vi "Prompt for Step.vi"(8 "error in (no error)":errorcluster, 10 "Subpanel Ref":refnum<vi>, 11 "Step in":refnum<class "Step.lvclass">) -> (0 "error out":errorcluster, 3 "Step out":refnum<class "Step.lvclass">)   [LabVIEW 2020, in "MacroAssert.lvlib" / "Step.lvclass"]
doc: "Displays its own window into <B>Subpanel Ref</B> for the user to enter a macro step."
uses:
  Step.lvclass
  <vilib>/Utility/inputDevices.llb/closeMouse.vi
  Support/Get Control Reference by Label (0D STR).vi
  SubVIs/FaKI State Machine/FaKI State Machine.lvlib
  MacroAssert.lvlib
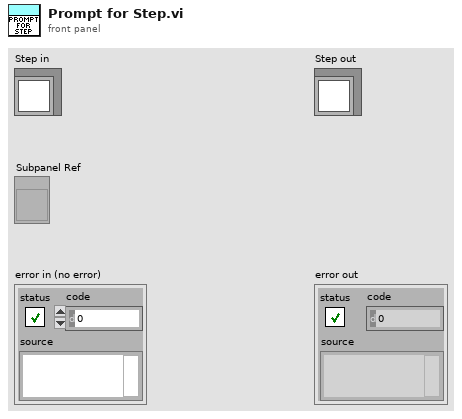
[diagram p1: front panel]
types:
  T1 = enum32{"Invalid", "Standard", "Closed", "Hidden", "Minimized", "Maximized"}
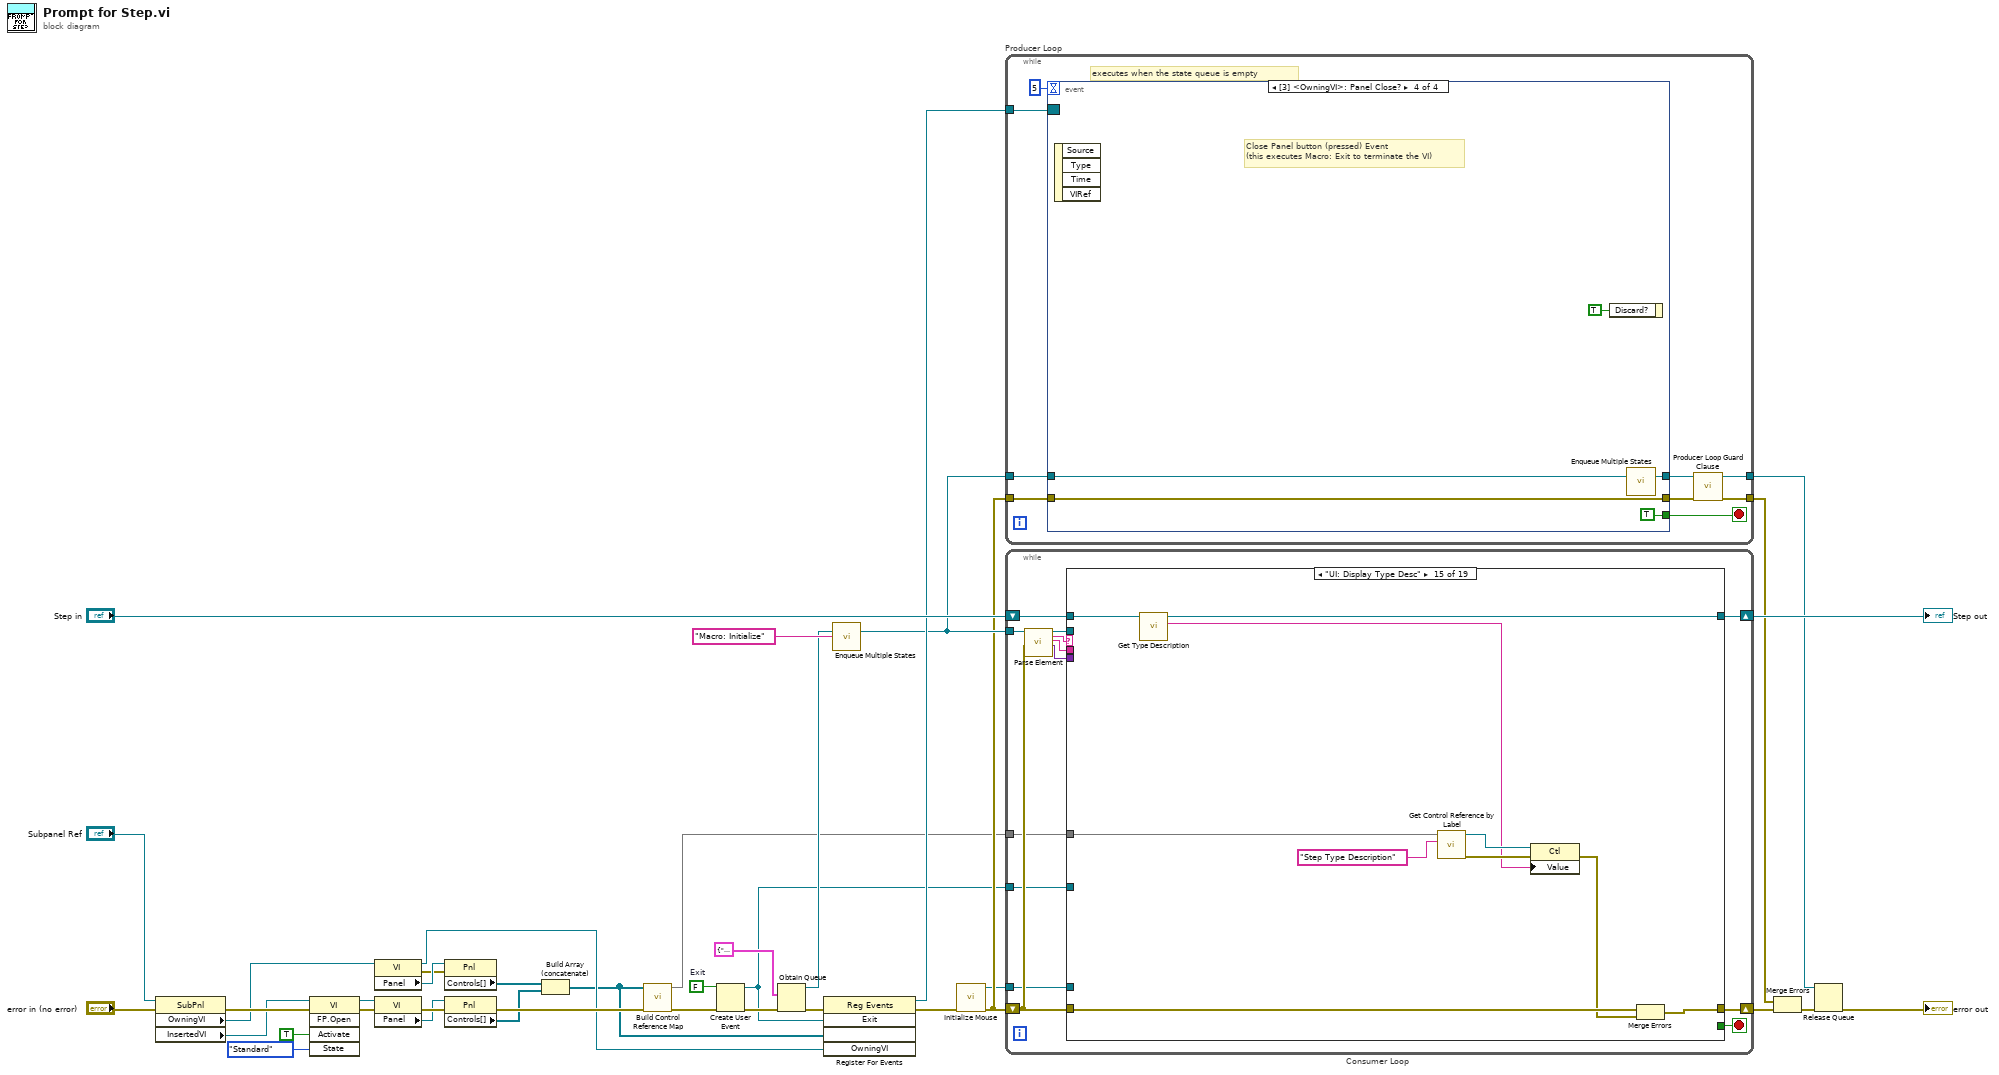
[diagram p0: block diagram]
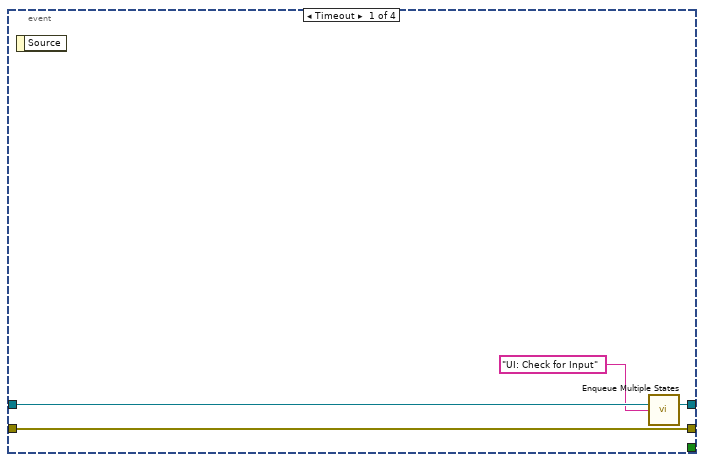
[diagram p2: hidden frame]
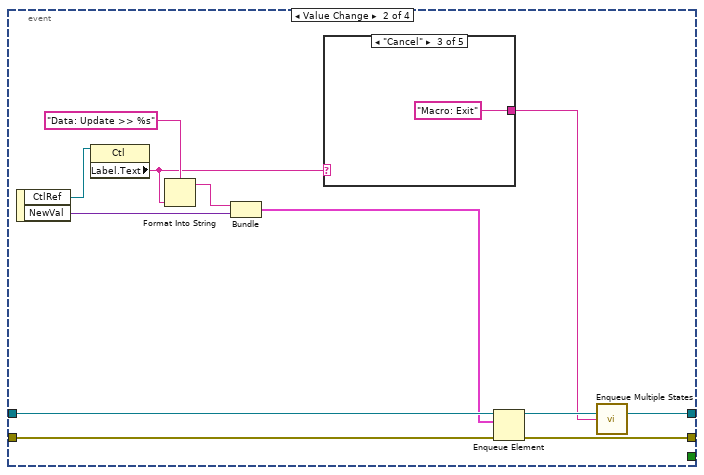
[diagram p3: hidden frame]
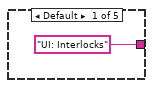
[diagram p4: hidden frame]
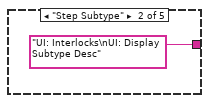
[diagram p5: hidden frame]
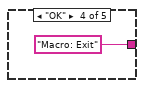
[diagram p6: hidden frame]
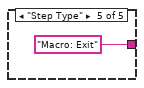
[diagram p7: hidden frame]
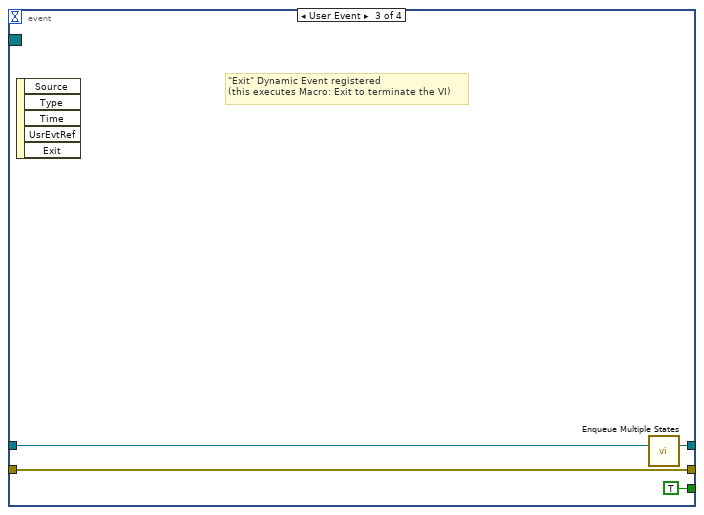
[diagram p8: hidden frame]
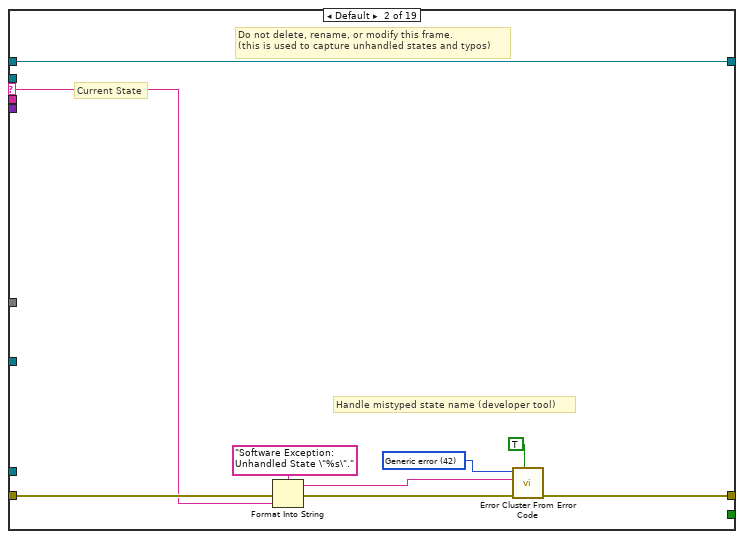
[diagram p10: hidden frame]
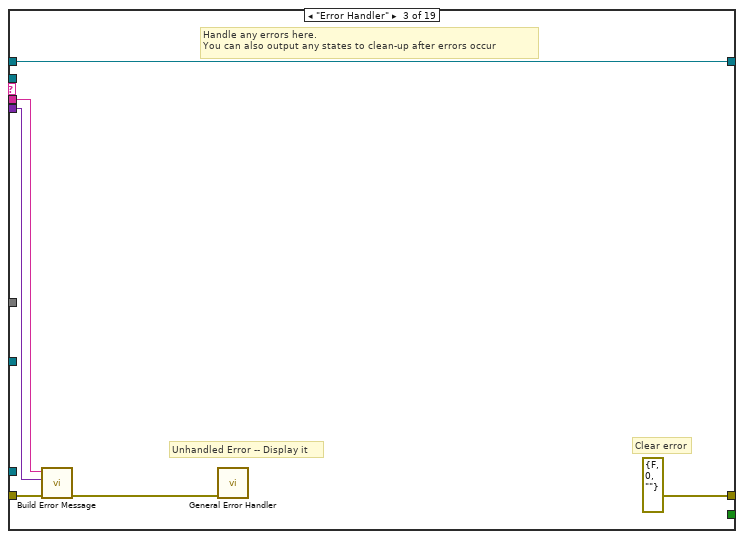
[diagram p11: hidden frame]
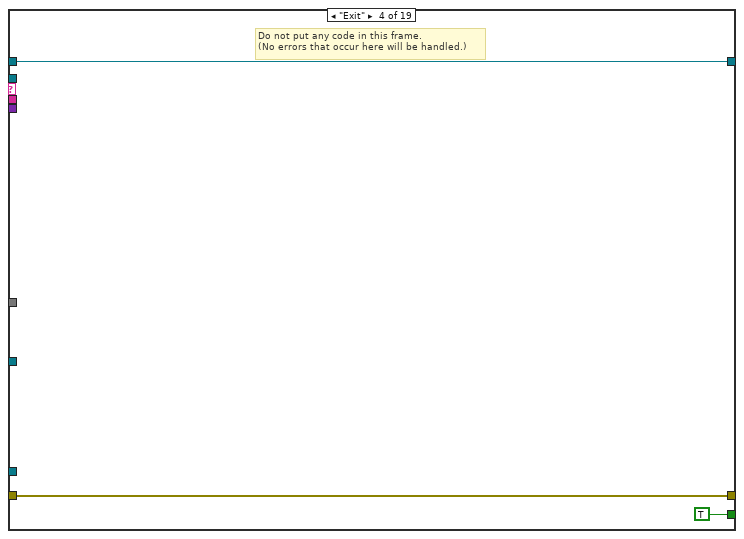
[diagram p12: hidden frame]
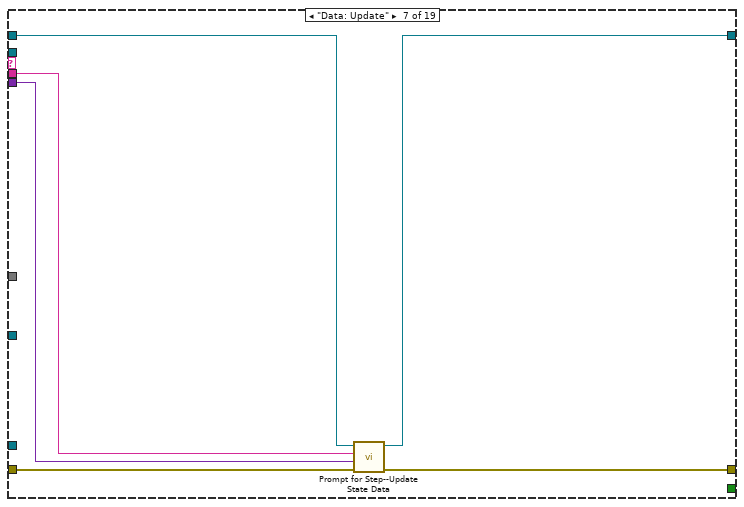
[diagram p15: hidden frame]
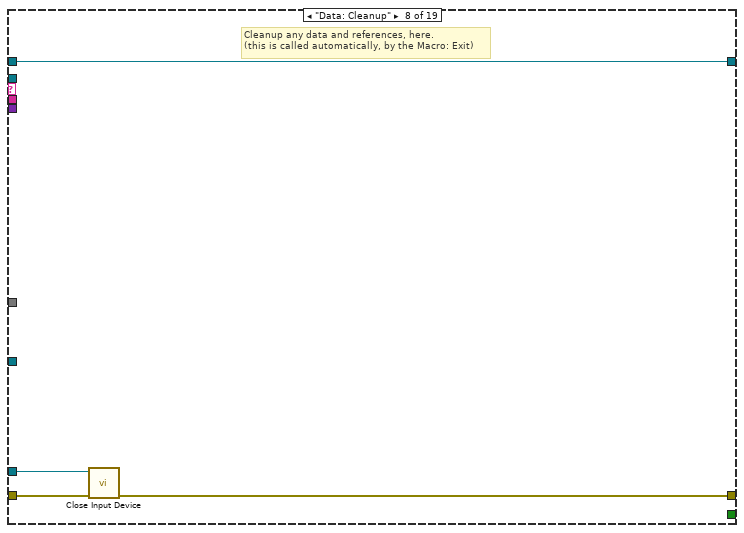
[diagram p16: hidden frame]
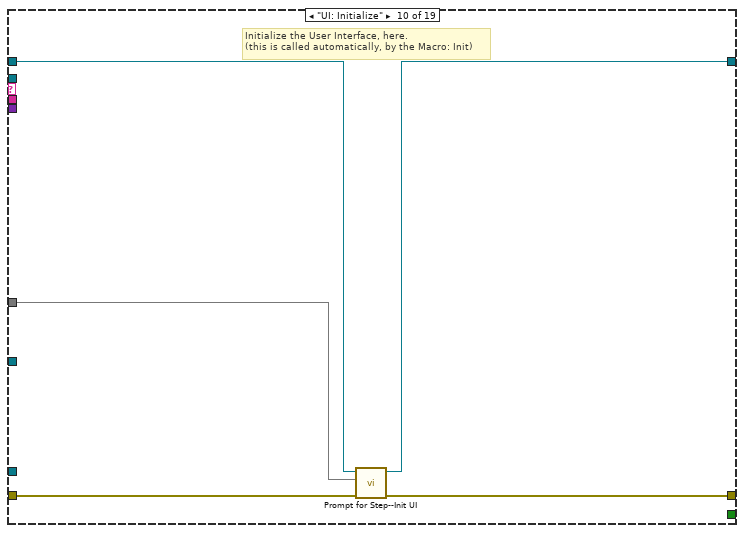
[diagram p18: hidden frame]
diagram:
  w7 = FALSE  # Exit
  n1 = property class="SubPnl"(reference="Subpanel Ref", error in="error in (no error)") -> (error out=w18:errorcluster, "OwningVI"=w10:refnum<vi>, "InsertedVI"=w11:refnum<vi>)  [unwired: 1 out]
  n2 = invoke class="VI" method="FP.Open"(reference=w11, error in=w18, "Activate"=TRUE, "State"=T1."Standard") -> (reference out=w16:refnum<vi>, error out=w17:errorcluster)  [unwired: 1 in, 3 out]
  n3 = property class="VI"(reference=w10) -> (reference out=w4:refnum<vi>, error out=w12:errorcluster, "Panel"=w13:refnum<vi>)  [unwired: 1 in]
  n4 = property class="VI"(reference=w16, error in=w17) -> (error out=w15:errorcluster, "Panel"=w14:refnum<vi>)  [unwired: 1 out]
  n5 = property class="Pnl"(reference=w13, error in=w12) -> ("Controls[]"=w9:refnum<vi>[])  [unwired: 2 out]
  n6 = property class="Pnl"(reference=w14, error in=w15) -> (error out=w39:errorcluster, "Controls[]"=w8:refnum<vi>[])  [unwired: 1 out]
  n7 = Build Array (concatenate)(w9, w8) -> (w3:refnum<vi>[])
  n8 = call "Build Control Reference Map.vi"("error in (no error)"=w39, "Control Refs"=w3) -> ("error out"=w2:errorcluster, "Control Ref Map"=w1:map{string, refnum<vi>})  [unwired: 8 in]
  n9 = Create User Event(user event datatype=w7, error in=w2) -> (user event=w5:refnum<user-event>, error out=w6:errorcluster)
  n10 = Obtain Queue(element data type=cluster{"State >> Arg":string, "Data":variant} {"State >> Arg"="", "Data"=variant}, error in (no error)=w6) -> (queue out=w27:refnum<queue>, error out=w34:errorcluster)  [unwired: 3 in, 1 out]
  n11 = register-events(error in=w34, w5, w3, w4) -> (reference out=w29:refnum<event-registration>, error out=w24:errorcluster)  [unwired: 1 in]
  n12 = call "Enqueue Multiple States.vi"("queue in"=w27, "State(s) at Back"="Macro: Initialize") -> ("queue out"=w25:refnum<queue>)  [unwired: 13 in]
  n13 = call <vilib>:"Initialize Mouse.vi"("error in (no error)"=w24) -> ("error out"=w23:errorcluster, "device ID"=w22:refnum<k1>)  [unwired: 9 in]
  n14 = while "Producer Loop" {
    tunnel: w29 -> [w40]
    tunnel: w25 -> [w46]
    tunnel: [w41] -> w30
    tunnel: w23 -> [w48]
    tunnel: [w43] -> w32
    stop <- w45 stop-if-true
    # "executes when the state queue is empty"
    n15 = event shown="[3] <OwningVI>: Panel Close?" {
      selector: w40 -> [_ _ _ _]
      dyn-events: _ -> [_ _ _ _]
      timeout: 5 ("Timeout") -> [_ _ _ _]
      tunnel: [w50 w60 w73 w78] -> w44
      tunnel: w48 -> [w50 w61 w73 w78]
      tunnel: w46 -> [w51 w54 w72 w77]
      tunnel: [w52 w56 w71 w76] -> w42
      tunnel: [_ _ TRUE TRUE] -> w45
      event Timeout {
        n16 = event-data() -> ()  [unwired: 1 in, 1 out]
        n17 = call "Enqueue Multiple States.vi"("queue in"=w51, "State(s) at Back"="UI: Check for Input") -> ("queue out"=w52:refnum<queue>)  [unwired: 13 in]
      }
      event Value Change {
        n18 = event-data() -> ("CtlRef"=w59:refnum<vi>, "NewVal"=w58:variant)  [unwired: 1 in]
        n19 = property class="Ctl"(reference=w59) -> ("Label.Text"=w62:string)  [unwired: 1 in, 2 out]
        n20 = Format Into String(format string="Data: Update >> %s", w62) -> (resulting string=w63:string)  [unwired: 2 in, 1 out]
        n21 = Bundle(w63, "NewVal"=w58) -> (w53:cluster{string, "NewVal":variant})  [unwired: 1 in]
        n22 = case shown="\"Cancel\"" w62 {
          tunnel: ["UI: Interlocks" ("string") "UI: Interlocks\nUI: Display Subtype Desc" ("string") "Macro: Exit" ("string") "Macro: Exit" ("string") "Macro: Exit" ("string")] -> w55
          frame Default {
          }
          frame "Step Subtype" {
          }
          frame "Cancel" {
          }
          frame "OK" {
          }
          frame "Step Type" {
          }
        }
        n23 = Enqueue Element(queue=w54, element=w53, error in (no error)=w61) -> (queue out=w57:refnum<queue>, error out=w60:errorcluster)  [unwired: 1 in, 1 out]
        n24 = call "Enqueue Multiple States.vi"("queue in"=w57, "State(s) at Back"=w55) -> ("queue out"=w56:refnum<queue>)  [unwired: 13 in]
      }
      event User Event {
        # "\"Exit\" Dynamic Event registered\n(this executes Macro: Exit to terminate the VI)"
        n25 = event-data() -> ()  [unwired: 1 in, 5 out]
        n26 = call "Enqueue Multiple States.vi"("queue in"=w72) -> ("queue out"=w71:refnum<queue>)  [unwired: 14 in]
      }
      event Panel Close? {
        # "Close Panel button (pressed) Event\n(this executes Macro: Exit to terminate the VI)"
        n27 = event-data() -> ()  [unwired: 1 in, 4 out]
        n28 = event-data("Discard?"=TRUE) -> ()  [unwired: 1 in, 1 out]
        n29 = call "Enqueue Multiple States.vi"("queue in"=w77) -> ("queue out"=w76:refnum<queue>)  [unwired: 14 in]
      }
    }
    n30 = call "Producer Loop Guard Clause.vi"("error in (no error)"=w44, "queue in"=w42) -> ("error out"=w43:errorcluster, "queue out"=w41:refnum<queue>)  [unwired: 8 in]
  }
  n31 = while "Consumer Loop" {
    shift-right: [w88] -> w36
    shift-left: "Step in" -> [w87]
    shift-right: [w91] -> w33
    shift-left: w23 -> [w90]
    tunnel: w25 -> [w86]
    tunnel: w5 -> [w81]
    tunnel: w1 -> [w80]
    tunnel: w22 -> [w79]
    stop <- w89 stop-if-true
    n32 = call "Parse Element.vi"("queue in"=w86, "error in (no error)"=w90) -> ("queue out"=w85:refnum<queue>, "State"=w84:string, "Arg"=w83:string, "Data"=w82:variant)  [unwired: 14 in]
    n33 = case shown="\"UI: Display Type Desc\"" w84 {
      selector: w84 -> [_ w94 _ _ _ _ _ _ _ _ _ _ _ _ _ _ _ _ _]
      tunnel: w85 -> [_ _ _ _ _ _ _ _ _ _ _ _ _ _ _ _ _ w175 w182]
      tunnel: w83 -> [_ _ w103 _ _ _ w116 _ _ _ _ _ _ w143 _ _ _ _ _]
      tunnel: w87 -> [w92 w96 w107 w110 w112 w114 w118 w125 w126 w130 w133 w135 w140 w144 w159 w171 w172 w176 w183]
      tunnel: [w93 w101 errorcluster {"status"=FALSE, "code"=0, "source"=""} ("error out") w111 w113 w115 w120 w122 w127 w131 w134 w136 w141 w145 w157 w166 w173 w177 w180] -> w91
      tunnel: w90 -> [w93 w100 w106 w111 w113 w115 w121 w124 w127 w132 w134 w136 w142 w146 w158 w169 w173 w177 w184]
      tunnel: [_ _ _ TRUE _ _ _ _ _ _ _ _ _ _ _ _ _ _ _] -> w89
      tunnel: [w92 w96 w107 w110 w112 w114 w119 w125 w126 w129 w133 w135 w139 w144 w152 w170 w172 w176 w183] -> w88
      tunnel: w82 -> [_ _ w104 _ _ _ w117 _ _ _ _ _ _ _ _ _ _ _ _]
      tunnel: w81 -> [_ _ _ _ _ _ _ _ _ _ _ _ _ _ _ _ _ _ w179]
      tunnel: w80 -> [_ _ _ _ _ _ _ _ _ w128 _ _ w137 _ w154 w163 _ _ _]
      tunnel: w79 -> [_ _ _ _ _ _ _ w123 _ _ _ _ w138 _ _ _ _ _ _]
      frame "---------- Core ----------" {
        # "Do not put any code in this frame.\n(it is a separator no-op)"
      }
      frame Default {
        w98 = 42 items=["No error", "Argument error", "Memory is full", "Out of zone", "End of file", "File already open", "Generic file I/O error", "File not found", "File permission error", "Disk is full", "Duplicate path", "Too many files open", "System feature not enabled", "Resource file not found", "Cannot add resource", "Resource not found", "Image not found", "Image memory error", "Pen does not exist", "Config type invalid", "Config token not found", "Config parse error", "Config memory error", "Bad external code format", "Bad external code offset", "External code not present", "Null window", "Destroy window error", "Null menu", "Print aborted", "Bad print record", "Print driver error", "Windows error during printing", "Memory error during printing", "Print dialog error", "Generic print error", "Invalid device refnum", "Device not found", "Device parameter error", "Device unit error", "Cannot open device", "Device call aborted", "Generic error", "Cancelled by user", "Object ID too low", "Object ID too high", "Object not in heap", "Unknown heap", "Unknown object (invalid DefProc)", "Unknown object (DefProc not in table)", "Message out of range", "Invalid (null) method", "Unknown message", "Manager call not supported", "Bad address", "Network operation in progress", "Network operation timed out", "Connection is busy", "Network attribute not supported", "Network error", "Address in use", "System out of memory", "Connection aborted", "Connection refused", "Not connected", "Already connected", "Connection closed", "Initialization error (interapplication manager)", "Bad occurrence", "Wait on unbound occurrence handler", "Occurrence queue overflow", "Datalog type conflict", "Unused", "Unrecognized type (interapplication manager)", "Memory corrupt", "Failed to make temporary DLL", "Old CIN version", "Drag socket not found", "Failed to load drop-object", "Failed to register OLE object", "Failed to release OLE object", "Format specifier type mismatch", "Unknown format specifier", "Too few format specifiers", "Too many format specifiers", "Scan failed", "Newer CIN version", "Error converting to variant", "Runtime menu error", "Password tampered", "Variant attribute not found", "Incompatible variant data type", "Event data is not available", "Event Store is not present", "Occurrence is not found", "Event Queue is not created", "Event info is not available", "Refnum passed is NULL", "Error retrieving Class GUID", "Error retrieving CoClass GUID", "Error retrieving TypeLib GUID.", "Bad built application magic bytes.", "Specific driver is different from the specific driver associated with the Logical Name.", "There is no session opened to the class driver.", "Max Error", "MAX - Error with config objects", "MAX - Error loading configuration", "MAX - Group not supported"]
        # "Current State"
        # "Do not delete, rename, or modify this frame.\n(this is used to capture unhandled states and typos)"
        # "Handle mistyped state name (developer tool)"
        n34 = Format Into String(format string="Software Exception: Unhandled State \"%s\"." ("message"), error in=w100, w94) -> (resulting string=w97:string, error out=w102:errorcluster)  [unwired: 1 in]
        n35 = call <vilib>:"Error Cluster From Error Code.vi"("show call chain? (False)"=TRUE, "error in (no error)"=w102, "error message (\"\")"=w97, "error code (0)"=w98) -> ("error out"=w101:errorcluster)  [unwired: 5 in]
      }
      frame "Error Handler" {
        # "Unhandled Error -- Display it"
        # "Handle any errors here.\nYou can also output any states to clean-up after errors occur"
        # "Clear error"
        n36 = call "Build Error Message.vi"("error in (no error)"=w106, "Data"=w104, "Arg"=w103) -> ("error out"=w105:errorcluster)  [unwired: 8 in]
        n37 = call <vilib>:"General Error Handler.vi"("error in (no error)"=w105) -> ()  [unwired: 10 in, 5 out]
      }
      frame "Exit" {
        # "Do not put any code in this frame.\n(No errors that occur here will be handled.)"
      }
      frame "---------- Data ----------" {
        # "Do not put any code in this frame.\n(It is a separator no-op. You can make a copy of this frame to create a new Data frame)"
      }
      frame "Data: Initialize" {
        # "Initialize the shift-register data, here."
      }
      frame "Data: Update" {
        n38 = call-dynamic "Prompt for Step--Update State Data.vi"("error in (no error)"=w121, "Data"=w117, "Argument"=w116, "Step in"=w118) -> ("error out"=w120:errorcluster, "Step out"=w119:refnum<class "Step.lvclass">)  [unwired: 6 in]
      }
      frame "Data: Cleanup" {
        # "Cleanup any data and references, here.\n(this is called automatically, by the Macro: Exit)"
        n39 = call-poly <vilib>:"Close Input Device.vi"("error in (no error)"=w124, "device ID"=w123) -> ("error out"=w122:errorcluster)  [unwired: 8 in]
      }
      frame "---------- UI ----------" {
        # "Do not put any code in this frame.\n(It is a separator no-op. You can make a copy of this frame to create a new UI frame)"
      }
      frame "UI: Initialize" {
        # "Initialize the User Interface, here.\n(this is called automatically, by the Macro: Init)"
        n40 = call-dynamic "Prompt for Step--Init UI.vi"("error in (no error)"=w132, "Control Ref Map"=w128, "Step in"=w130) -> ("error out"=w131:errorcluster, "Step out"=w129:refnum<class "Step.lvclass">)  [unwired: 7 in]
      }
      frame "UI: Uninitialize" {
        # "Uninitialize the User Interface, here.\n(this is called automatically, by the Macro: Exit)"
      }
      frame "UI: Interlocks" {
      }
      frame "UI: Check for Input" {
        n41 = call-dynamic "Prompt for Step--Check for Input.vi"("error in (no error)"=w142, "Control Ref Map"=w137, "Mouse Ref"=w138, "Step in"=w140) -> ("error out"=w141:errorcluster, "Step out"=w139:refnum<class "Step.lvclass">)  [unwired: 6 in]
      }
      frame "UI: Cursor Set" {
        # "Argument"
        # "Set and Unset Cursor Busy.\n(Usage: \"UI: Cursor Set >> Busy|Idle\")"
        n42 = case shown="\"Idle\", Default" w143 {
          tunnel: w146 -> [w148 w150]
          tunnel: [w147 w149] -> w145
          frame "Idle", Default {
            n43 = call <vilib>:"Unset Busy.vi"("error in (no error)"=w148) -> ("error out"=w147:errorcluster)  [unwired: 10 in]
          }
          frame "Busy" {
            n44 = call <vilib>:"Set Busy.vi"("error in (no error)"=w150) -> ("error out"=w149:errorcluster)  [unwired: 9 in, 1 out]
          }
        }
      }
      frame "UI: Display Type Desc" {
        n45 = call "Get Type Description.vi"("Step in"=w159) -> ("Type Description"=w151:string, "Step out"=w152:refnum<class "Step.lvclass">)  [unwired: 8 in, 1 out]
        n46 = call-poly "Get Control Reference by Label.vi"("Control Name"="Step Type Description", "Control Ref Map"=w154) -> ("error out"=w155:errorcluster, "Control Ref"=w160:refnum<vi>)  [unwired: 7 in, 1 out]
        n47 = property class="Ctl"(reference=w160, error in=w155, "Value"=w151) -> (error out=w156:errorcluster)  [unwired: 1 out]
        n48 = Merge Errors(w158, w156) -> (w157:errorcluster)
      }
      frame "UI: Display Subtype Desc" {
        n49 = call-dynamic "Get Subtype Description.vi"("error in (no error)"=w169, "Step in"=w171) -> ("error out"=w168:errorcluster, "Subtype Description"=w167:string, "Step out"=w170:refnum<class "Step.lvclass">)  [unwired: 7 in]
        n50 = call-poly "Get Control Reference by Label.vi"("Control Name"="Subtype Description", "Control Ref Map"=w163) -> ("error out"=w164:errorcluster, "Control Ref"=w161:refnum<vi>)  [unwired: 7 in, 1 out]
        n51 = property class="Ctl"(reference=w161, error in=w164, "Value"=w167) -> (error out=w165:errorcluster)  [unwired: 1 out]
        n52 = Merge Errors(w168, w165) -> (w166:errorcluster)
      }
      frame "---------- Macro ----------" {
        # "Do not put any code in this frame.\n(It is a separator no-op. You can make a copy of this frame to create a new Macro frame)"
      }
      frame "Macro: Initialize" {
        # "Initialization Macro\n(This is called once, when the VI starts)"
        n53 = call "Enqueue Multiple States.vi"("State(s) at Front"="Data: Initialize\nUI: Initialize\nUI: Display Type Desc\nUI: Display Subtype Desc", "queue in"=w175) -> ()  [unwired: 13 in, 1 out]
      }
      frame "Macro: Exit" {
        # "Exit Macro\n(This is called once, when the VI exits)"
        n54 = Generate User Event(user event=w179, event data cluster=FALSE ("event data"), error in=w184) -> (error out=w180:errorcluster)  [unwired: 1 in, 1 out]
        n55 = call "Enqueue Multiple States.vi"("State(s) at Front"="UI: Uninitialize\nData: Cleanup\nExit", "queue in"=w182) -> ()  [unwired: 13 in, 1 out]
      }
    }
  }
  "Step out" <- w36
  n56 = Merge Errors(w32, w33) -> (w31:errorcluster)
  n57 = Release Queue(queue=w30, error in (no error)=w31) -> (error out=→"error out":errorcluster)  [unwired: 1 in, 2 out]
